vi "getTaskInfo.vi"(8 "error in (no error)":errorcluster, 11 "VGS_RemoteControlClient in":refnum<class "VGS_RemoteControlClient.lvclass">) -> (0 "error out":errorcluster, 1 "getTaskInfo":refnum<k24>, 2 "Task Info":T1, 3 "VGS_RemoteControlClient out":refnum<class "VGS_RemoteControlClient.lvclass">)   [LabVIEW 2022 SP3, in "LV_VGS.lvlib" / "VGS_RemoteControlClient.lvclass"]
doc: "<B>Get information about the current task on a VGStudio (MAX) instance. </B>\n\nThis method gets the current task information of a VGStudio (MAX) instance. If the application is Idle mode then the method returns a default TaskInfo instance. \n\nDefault values are:\n\nti.Description = \"\";\nti.DetailedDescription = \"\";\nti.Diagnostics = \"\";\nti.ProgressPercentage = 0.0f;\nti.Timestamp = 0.0f;\n\nParameters\nhandle A valid remote handle. \n\nEmit error RemoteControlServiceIsNotAvailableException if the remote control service doesn't run. \nEmit error GenericRemoteControlErrorException if an internal error occurs.\nEmit error InvalidRemoteHandleException if the remote handle is not valid."
uses:
  VGS_RemoteControlClient.lvclass
  C:/Users/Andrey/Desktop/hajo/LV_VGS/vgs_project.dll
  vgs_project.dll
  typedefs/TaskInfo.ctl
  VGS_RemoteControlClient.lvclass/VGS_RemoteControlClient.ctl
  LV_VGS.lvlib
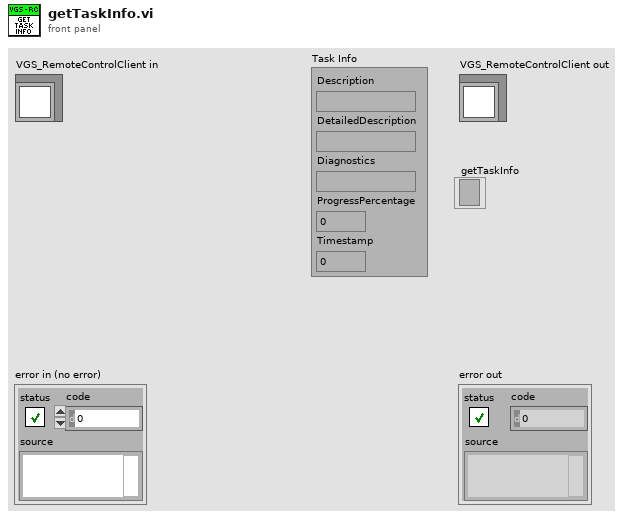
[diagram p1: front panel]
types:
  T1 = typedef "LV_VGS.lvlib/TaskInfo.ctl" = cluster{"Description":string, "DetailedDescription":string, "Diagnostics":string, "ProgressPercentage":sgl, "Timestamp":dbl}
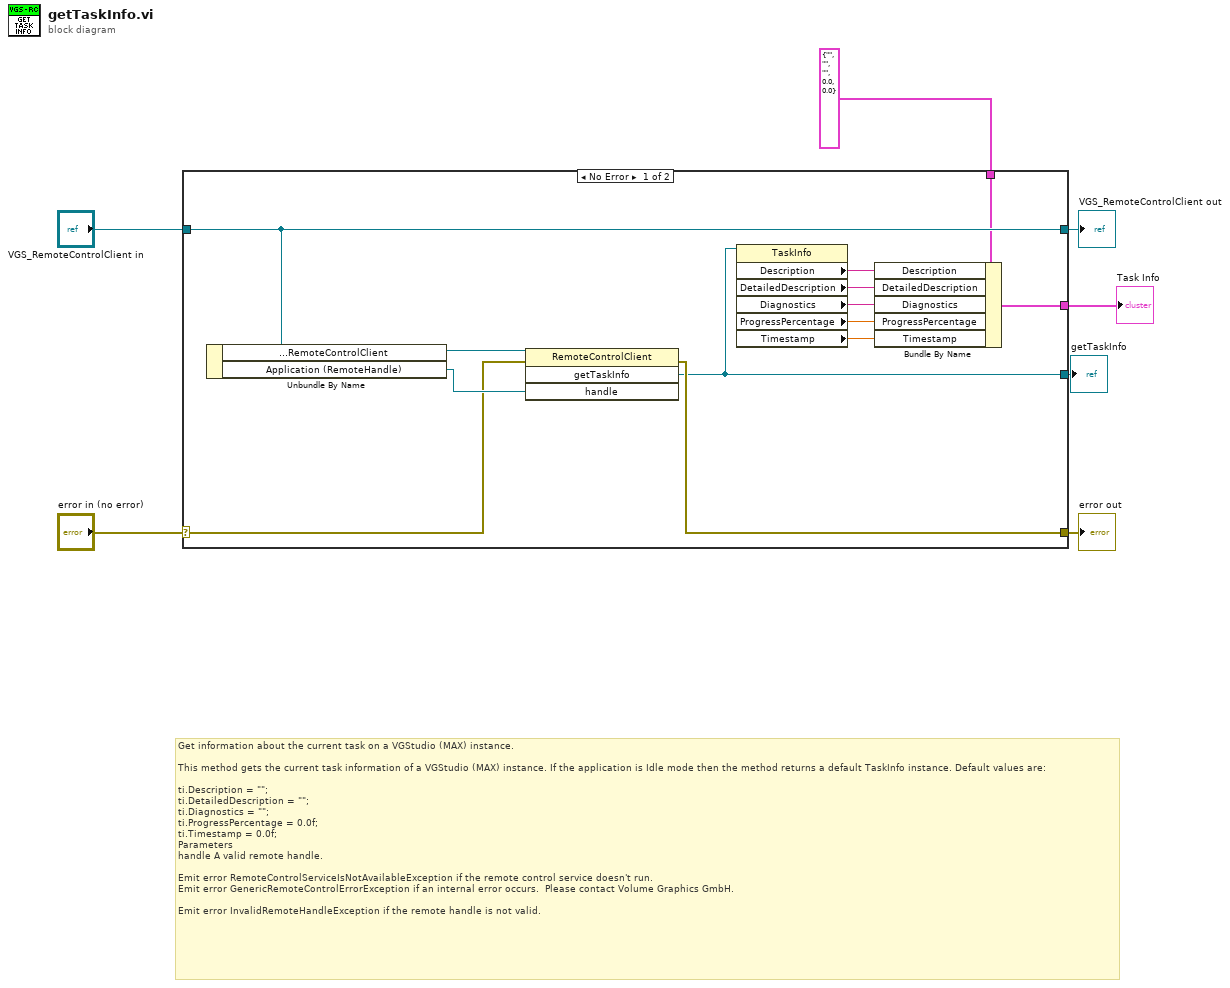
[diagram p0: block diagram]
diagram:
  # "Get information about the current task on a VGStudio (MAX) instance. \n\nThis method gets the current task information of a VGStudio (MAX) instance. If the application is Idle mode then the method returns a default TaskInfo instance. Default values are:\n\nti.Description = \"\";\nti.DetailedDescription = \"\";\nti.Diagnostics = \"\";\nti.ProgressPercentage = 0.0f;\nti.Timestamp = 0.0f;\nParameters\nhandle A valid remote handle. \n\nEmit error RemoteControlServiceIsNotAvailableException if the remote control service doesn't run. \nEmit error GenericRemoteControlErrorException if an internal error occurs.  Please contact Volume Graphics GmbH.  \n\nEmit error InvalidRemoteHandleException if the remote handle is not valid."
  n1 = case shown="No Error" "error in (no error)" {
    selector: "error in (no error)" -> [w17 w22]
    tunnel: [w16 w22] -> w6
    tunnel: [w20 w21] -> w4
    tunnel: "VGS_RemoteControlClient in" -> [w20 w21]
    tunnel: [w15 _] -> w3
    tunnel: T1 {"Description"="", "DetailedDescription"="", "Diagnostics"="", "ProgressPercentage"=0.0, "Timestamp"=0.0} ("TaskInfo") -> [w14 _]
    tunnel: [w8 _] -> w1
    frame No Error {
      n2 = Unbundle By Name(w20) -> ("VGS.Project.Interop.RemoteControlClient"=w19:refnum<k24>, "Application (RemoteHandle)"=w18:refnum<k24>)
      n3 = invoke class="RemoteControlClient" method="getTaskInfo"(reference=w19, error in=w17, "handle"=w18) -> (error out=w16:errorcluster, "getTaskInfo"=w15:refnum<k24>)  [unwired: 1 in, 2 out]
      n4 = property class="TaskInfo"(reference=w15) -> ("Description"=w13:string, "DetailedDescription"=w12:string, "Diagnostics"=w11:string, "ProgressPercentage"=w10:sgl, "Timestamp"=w9:dbl)  [unwired: 1 in, 2 out]
      n5 = Bundle By Name(cluster=w14, "Description"=w13, "DetailedDescription"=w12, "Diagnostics"=w11, "ProgressPercentage"=w10, "Timestamp"=w9) -> (w8:T1)
    }
    frame Error {
    }
  }
  "error out" <- w6
  "VGS_RemoteControlClient out" <- w4
  "getTaskInfo" <- w3
  "Task Info" <- w1
